vi "Rotation3d_Create_InitialFinalVector.vi"(9 "Final Vector":T1, 11 "Initial Vector":T1) -> (3 "ROTATION3D":T2={"Q_quaternion"={"R"=1.0, "V"=[0.0, 0.0, 0.0]}})   [LabVIEW 2019, in "Trajectory_Library.lvlib"]
doc: "Constructs a Rotation3d that rotates the initial vector onto the final vector.\n\nThis is useful for turning a 3D vector (final) into an orientation relative to a coordinate system vector (initial).\n\nParmeters:\n - initial -- The initial vector.\n - last -- .The final vector\n\nReturns\n - rotation data structure"
uses:
  Trajectory_Library.lvlib
  <vilib>/Analysis/NI_AALPro.lvlib
  <vilib>/Analysis/7linalg.llb/Real QR Decomposition.vi
  TypeDef/QUATERNION.ctl
  TypeDef/ROTATION3D.ctl
  <vilib>/Analysis/Matrix/Datatypes/RealMatrix.ctl
  <vilib>/Analysis/Matrix/NI_Matrix.lvlib
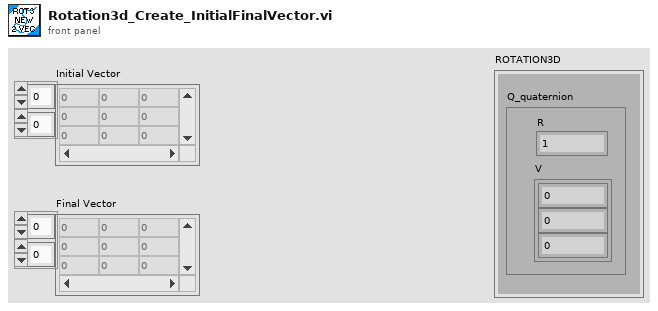
[diagram p1: front panel]
types:
  T1 = typedef "NI_Matrix.lvlib/RealMatrix.ctl" = dbl[][]
  T2 = typedef "Trajectory_Library.lvlib/ROTATION3D.ctl" = cluster{"Q_quaternion":T3}
  T3 = typedef "Trajectory_Library.lvlib/QUATERNION.ctl" = cluster{"R":dbl, "V":dbl[]}
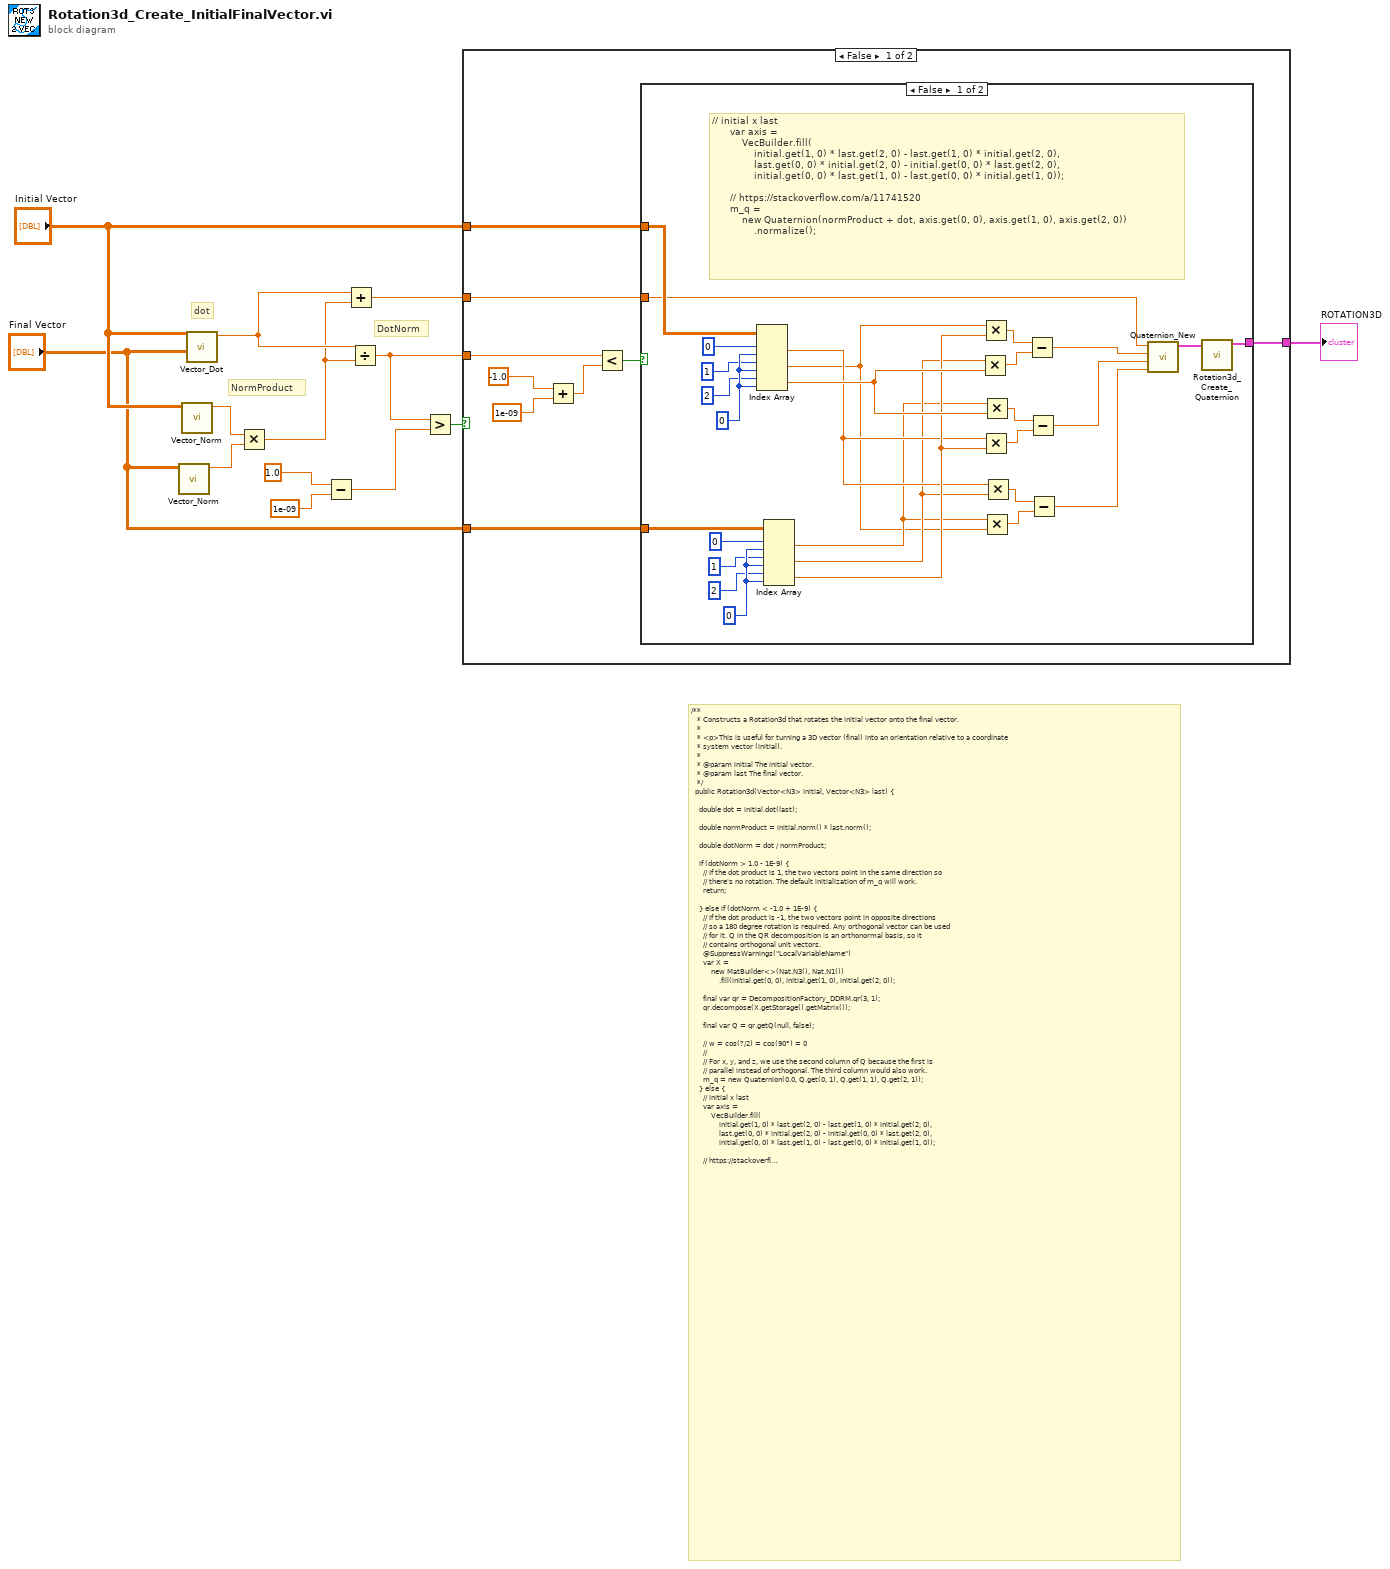
[diagram p0: block diagram]
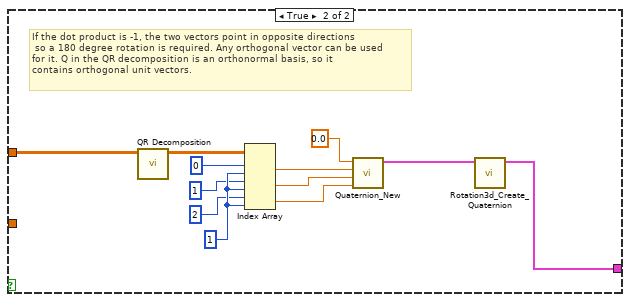
[diagram p2: hidden frame]
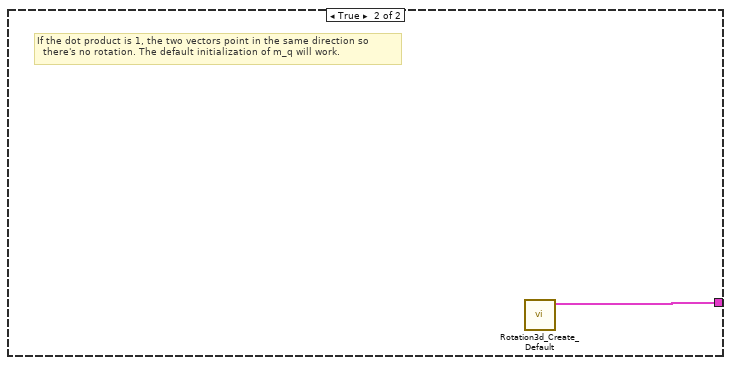
[diagram p3: hidden frame]
diagram:
  # "DotNorm"
  # "NormProduct"
  # "dot"
  # "/**\n   * Constructs a Rotation3d that rotates the initial vector onto the final vector.\n   *\n   * <p>This is useful for turning a 3D vector (final) into an orientation relative to a coordinate\n   * system vector (initial).\n   *\n   * @param initial The initial vector.\n   * @param last The final vector.\n   */\n  public Rotation3d(Vector<N3> initial, Vector<N3> last) {\n\n    double dot = initial.dot(last);\n\n    double normProduct = initial.norm() * last.norm();\n\n    double dotNorm = dot / normProduct;\n\n    if (dotNorm > 1.0 - 1E-9) {\n      // If the dot product is 1, the two vectors point in the same direction so\n      // there's no rotation. The default initialization of m_q will work.\n      return;\n\n    } else if (dotNorm < -1.0 + 1E-9) {\n      // If the dot product is -1, the two vectors point in opposite directions\n      // so a 180 degree rotation is required. Any orthogonal vector can be used\n      // for it. Q in the QR decomposition is an orthonormal basis, so it\n      // contains orthogonal unit vectors.\n      @SuppressWarnings(\"LocalVariableName\")\n      var X =\n          new MatBuilder<>(Nat.N3(), Nat.N1())\n              .fill(initial.get(0, 0), initial.get(1, 0), initial.get(2, 0));\n\n      final var qr = DecompositionFactory_DDRM.qr(3, 1);\n      qr.decompose(X.getStorage().getMatrix());\n\n      final var Q = qr.getQ(null, false);\n\n      // w = cos(?/2) = cos(90°) = 0\n      //\n      // For x, y, and z, we use the second column of Q because the first is\n      // parallel instead of orthogonal. The third column would also work.\n      m_q = new Quaternion(0.0, Q.get(0, 1), Q.get(1, 1), Q.get(2, 1));\n    } else {\n      // initial x last\n      var axis =\n          VecBuilder.fill(\n              initial.get(1, 0) * last.get(2, 0) - last.get(1, 0) * initial.get(2, 0),\n              last.get(0, 0) * initial.get(2, 0) - initial.get(0, 0) * last.get(2, 0),\n              initial.get(0, 0) * last.get(1, 0) - last.get(0, 0) * initial.get(1, 0));\n\n      // https://stackoverflow.com/a/11741520\n      m_q =\n          new Quaternion(normProduct + dot, axis.get(0, 0), axis.get(1, 0), axis.get(2, 0))\n              .normalize();\n    }\n  }"
  n1 = call "Vector_Norm.vi"("Input Vector"="Final Vector") -> ("norm"=w12:dbl)  [unwired: 10 in]
  n2 = call "Vector_Norm.vi"("Input Vector"="Initial Vector") -> ("norm"=w13:dbl)  [unwired: 10 in]
  n3 = call "Vector_Dot.vi"("Input Vector 2"="Final Vector", "Input Vector 1"="Initial Vector") -> ("dot product"=w3:dbl)  [unwired: 9 in]
  n4 = Multiply(x=w13, y=w12) -> (x*y=w2:dbl)
  n5 = Subtract(x=1.0, y=1e-09) -> (x-y=w9:dbl)
  n6 = Add(x=w3, y=w2) -> (x+y=w1:dbl)
  n7 = Divide(x=w3, y=w2) -> (x/y=w6:dbl)
  n8 = Greater?(x=w6, y=w9) -> (0:w8:bool)
  n9 = case shown="False" w8 {
    tunnel: [w16 w63] -> w7
    tunnel: w6 -> [w20 _]
    tunnel: "Initial Vector" -> [w17 _]
    tunnel: "Final Vector" -> [w15 _]
    tunnel: w1 -> [w14 _]
    frame False {
      n10 = Add(x=-1.0, y=1e-09) -> (x+y=w19:dbl)
      n11 = Less?(x=w20, y=w19) -> (x < y?=w18:bool)
      n12 = case shown="False" w18 {
        tunnel: w17 -> [w46 w62]
        tunnel: [w23 w52] -> w16
        tunnel: w15 -> [w41 _]
        tunnel: w14 -> [w28 _]
        frame False {
          w44 = 0 ("index (col)")
          w49 = 0 ("index (col)")
          # "// initial x last\n      var axis =\n          VecBuilder.fill(\n              initial.get(1, 0) * last.get(2, 0) - last.get(1, 0) * initial.get(2, 0),\n              last.get(0, 0) * initial.get(2, 0) - initial.get(0, 0) * last.get(2, 0),\n              initial.get(0, 0) * last.get(1, 0) - last.get(0, 0) * initial.get(1, 0));\n\n      // https://stackoverflow.com/a/11741520\n      m_q =\n          new Quaternion(normProduct + dot, axis.get(0, 0), axis.get(1, 0), axis.get(2, 0))\n              .normalize();"
          n13 = Index Array(array=w46, index (row) #1=0 ("index (row)"), index (col) #1=w49, index (row) #2=1 ("index (row)"), index (col) #2=w49, index (row) #3=2 ("index (row)"), index (col) #3=w49) -> (element #1=w32:dbl, element #2=w29:dbl, element #3=w34:dbl)
          n14 = Index Array(array=w41, index (row) #1=0 ("index (row)"), index (col) #1=w44, index (row) #2=1 ("index (row)"), index (col) #2=w44, index (row) #3=2 ("index (row)"), index (col) #3=w44) -> (element #1=w30:dbl, element #2=w31:dbl, element #3=w33:dbl)
          n15 = Multiply(x=w31, y=w34) -> (x*y=w39:dbl)
          n16 = Multiply(x=w29, y=w33) -> (x*y=w40:dbl)
          n17 = Multiply(x=w32, y=w33) -> (x*y=w37:dbl)
          n18 = Multiply(x=w30, y=w34) -> (x*y=w38:dbl)
          n19 = Multiply(x=w30, y=w29) -> (x*y=w35:dbl)
          n20 = Multiply(x=w32, y=w31) -> (x*y=w36:dbl)
          n21 = Subtract(x=w40, y=w39) -> (x-y=w27:dbl)
          n22 = Subtract(x=w38, y=w37) -> (x-y=w26:dbl)
          n23 = Subtract(x=w36, y=w35) -> (x-y=w25:dbl)
          n24 = call "Quaternion_New.vi"("Z"=w25, "Y"=w26, "X"=w27, "W"=w28) -> ("out Quaternion"=w24:T3)  [unwired: 7 in]
          n25 = call "Rotation3d_Create_Quaternion.vi"("Quaternion"=w24) -> ("Rotation3d"=w23:T2)  [unwired: 10 in]
        }
        frame True {
          w59 = 1 ("index (col)")
          # "If the dot product is -1, the two vectors point in opposite directions\n so a 180 degree rotation is required. Any orthogonal vector can be used\nfor it. Q in the QR decomposition is an orthonormal basis, so it\ncontains orthogonal unit vectors."
          n26 = call-poly <vilib>:"QR Decomposition.vi"("A"=w62) -> ("Q"=w61:T1)  [unwired: 7 in, 3 out]
          n27 = Index Array(array=w61, index (row) #1=0 ("index (row)"), index (col) #1=w59, index (row) #2=1 ("index (row)"), index (col) #2=w59, index (row) #3=2 ("index (row)"), index (col) #3=w59) -> (element #1=w57:dbl, element #2=w54:dbl, element #3=w53:dbl)
          n28 = call "Quaternion_New.vi"("Z"=w53, "Y"=w54, "X"=w57, "W"=0.0) -> ("out Quaternion"=w51:T3)  [unwired: 7 in]
          n29 = call "Rotation3d_Create_Quaternion.vi"("Quaternion"=w51) -> ("Rotation3d"=w52:T2)  [unwired: 10 in]
        }
      }
    }
    frame True {
      # "If the dot product is 1, the two vectors point in the same direction so\n  there's no rotation. The default initialization of m_q will work."
      n30 = call "Rotation3d_Create_Default.vi"() -> ("ROTATION3D"=w63:T2)  [unwired: 11 in]
    }
  }
  "ROTATION3D" <- w7
